vi "AES_sci_idle.vi"   [LabVIEW 2016]
uses:
  Sci/SciShutt.lvclass
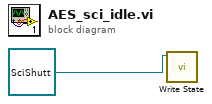
[diagram p0: block diagram]
diagram:
  n1 = call-dynamic "Write State.vi"("Shutter in"=refnum<class "SciShutt.lvclass"> refnum ("SciShutt.lvclass")) -> ()  [unwired: 9 in, 2 out]
